vi "Pack for gRPC.vi"(8 "error in":errorcluster, 9 "configuration / results":enum16{"Configuration", "Results"}(ring), 10 "data value":variant, 11 "measurement customizations in":refnum<class "Measurement Plugin.lvclass">) -> (0 "error out":errorcluster, 2 "any":T1, 3 "measurement customizations out":refnum<class "Measurement Plugin.lvclass">)   [LabVIEW 2021, in "Line Transient_Channel Ganging.lvlib" / "Measurement Plugin.lvclass"]
uses:
  Measurement Plugin.lvclass
  Measurement Plugin.lvclass/Measurement Plugin.ctl
  Measurement Configuration.ctl
  Line Transient_Channel Ganging.lvlib
  Measurement Results.ctl
  a6012965-5700-4384-8228-972e71b6560c.vi
  2eca732d-dbaa-43bf-a7dd-ede2da65bc1b.vi
  <vilib>/Plug-In SDKs/Measurements/Measurement Plugin Service/Measurement Plugin Service.lvclass
  C:/Program Files/National Instruments/LabVIEW 2021/vi.lib/Plug-In SDKs/Measurements/Measurement Plugin Service/Measurement Plugin Service.lvclass
  C:/pmic-labview/source/channel ganging/line transient channel ganging/Line Transient_Channel Ganging/Advanced/Measurement Plugin.lvclass
  <vilib>/gRPC/LabVIEW gRPC Library/Shared/Any.ctl
  <vilib>/gRPC/LabVIEW gRPC Library/grpc-lvsupport-release.lvlib
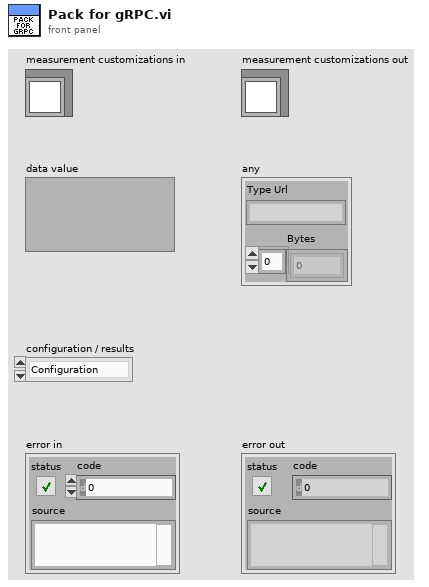
[diagram p1: front panel]
types:
  T1 = typedef "grpc-lvsupport-release.lvlib/Any.ctl" = cluster{"Type Url":string, "Bytes":u8[]}
  T2 = typedef "grpc-lvsupport-release.lvlib/grpcId.ctl" = u64
  T3 = typedef "Line Transient_Channel Ganging.lvlib/Measurement Configuration.ctl" = cluster{"Source master resource name":string, "Load master resource name":string, "Source slave resource names":string[], "Load slave resource names":string[], "Source system configuration":enum32{"Series", "Parallel", "Manual"}, "Source voltage level range":dbl, "Source limit symmetry":enum32{"Symmetric", "Asymmetric"}, "Source current limit range":dbl, "Source current limit low":dbl, "Source current limit high":dbl, "Source transient response":i32, "Source sense":i32, "Source voltage level 1":dbl, "Source sample rate":dbl, "Source voltage level 2":dbl, "Source voltage gain bandwidth":dbl, "Source voltage compensation frequency":dbl, "Source voltage pole-zero ratio":dbl, "Load system configuration":enum32{"Series", "Parallel", "Manual"}, "Load current level":dbl, "Load current level range":dbl, "Load limit symmetry":enum32{"Symmetric", "Asymmetric"}, "Load voltage limit range":dbl, "Load voltage limit low":dbl, "Load voltage limit high":dbl, "Load transient response":i32, "Load sense":i32, "DUT setup time":dbl, "Load current gain bandwidth":dbl, "Load current compensation frequency":dbl, "Load current pole-zero ratio":dbl, "Nominal output voltage":dbl, "Source time delay 1":dbl, "Source time delay 2":dbl, "Source pulse duration":dbl, "Source voltage falling slew rate":dbl, "Source voltage rising slew rate":dbl, "Scope resource name":string, "Scope output channel name":string, "Scope sample rate":dbl, "Scope probe attenuation":dbl, "Scope vertical range":dbl, "Scope vertical coupling":enum32{"AC", "DC"}, "Scope enable/disable":bool}
  T4 = typedef "Line Transient_Channel Ganging.lvlib/Measurement Results.ctl" = cluster{"Smu dt":dbl, "Load voltages":dbl[], "Source voltages":dbl[], "Scope amplitudes":dbl[], "Scope dt":dbl}
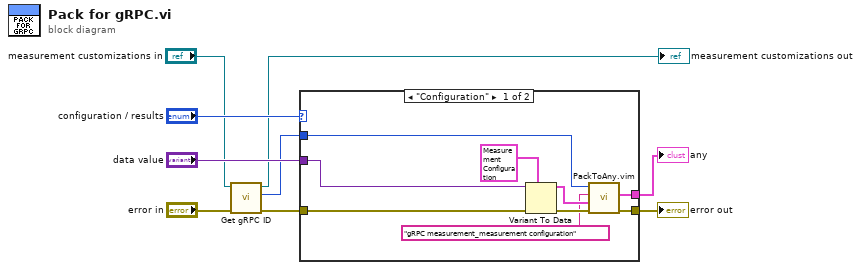
[diagram p0: block diagram]
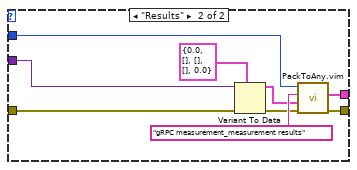
[diagram p2: hidden frame]
diagram:
  n1 = call <vilib>:"Get gRPC ID.vi"("error in"="error in", "measurement plugin service in"="measurement customizations in") -> ("error out"=w4:errorcluster, "gRPC ID"=w1:T2, "measurement plugin service out"=→"measurement customizations out":refnum<class "Measurement Plugin.lvclass">)  [unwired: 7 in]
  n2 = case shown="\"Configuration\"" "configuration / results" {
    tunnel: w4 -> [w18 w27]
    tunnel: "data value" -> [w17 w26]
    tunnel: w1 -> [w14 w22]
    tunnel: [w16 w24] -> w8
    tunnel: [w15 w23] -> w7
    frame "Configuration" {
      n3 = Variant To Data(error in=w18, type=T3 {"Source master resource name"="Lorem ipsum dolor sit", "Load master resource name"="", "Source slave resource names"=["", ""], "Load slave resource names"=[], "Source system configuration"=enum."Parallel", "Source voltage level range"=64.0, "Source limit symmetry"=enum."Asymmetric", "Source current limit range"=-32.0, "Source current limit low"=-64.0, "Source current limit high"=-64.0, "Source transient response"=1, "Source sense"=1, "Source voltage level 1"=1.0, "Source sample rate"=1.0, "Source voltage level 2"=14.0, "Source voltage gain bandwidth"=2000.0, "Source voltage compensation frequency"=3530.0, "Source voltage pole-zero ratio"=2.0, "Load system configuration"=enum."Parallel", "Load current level"=1.0, "Load current level range"=80.0, "Load limit symmetry"=enum."Symmetric", "Load voltage limit range"=6.0, "Load voltage limit low"=0.0, "Load voltage limit high"=inf, "Load transient response"=1038, "Load sense"=1009, "DUT setup time"=1.0, "Load current gain bandwidth"=14000.0, "Load current compensation frequency"=180000.0, "Load current pole-zero ratio"=0.3, "Nominal output voltage"=1.0, "Source time delay 1"=6.0, "Source time delay 2"=0.005, "Source pulse duration"=0.005, "Source voltage falling slew rate"=24.0, "Source voltage rising slew rate"=24.0, "Scope resource name"="", "Scope output channel name"="0", "Scope sample rate"=1800000.0, "Scope probe attenuation"=1.0, "Scope vertical range"=10.0, "Scope vertical coupling"=enum."DC", "Scope enable/disable"=TRUE} ("measurement configuration"), Variant=w17) -> (data=w13:T3, error out=w12:errorcluster)
      n4 = call "PackToAny.vim"("error in"=w12, "Data To Pack"=w13, "Message Type"="gRPC measurement_measurement configuration", "gRPCid in"=w14) -> ("error out"=w16:errorcluster, "Any"=w15:T1)  [unwired: 5 in, 1 out]
    }
    frame "Results" {
      n5 = Variant To Data(error in=w27, type=T4 {"Smu dt"=0.0, "Load voltages"=[], "Source voltages"=[], "Scope amplitudes"=[], "Scope dt"=0.0} ("Measurement Results"), Variant=w26) -> (data=w20:T4, error out=w19:errorcluster)
      n6 = call "PackToAny.vim"("error in"=w19, "Data To Pack"=w20, "Message Type"="gRPC measurement_measurement results", "gRPCid in"=w22) -> ("error out"=w24:errorcluster, "Any"=w23:T1)  [unwired: 5 in, 1 out]
    }
  }
  "error out" <- w8
  "any" <- w7
